vi "Load_LDA_Channel_Setup.vi"(1 "LDA Setup":T1[](array[typedef]) {"Fs" format="%#_pHz"; "syncDelay" format="%#_gms"; "Ch" min=0 step=1}, 2 "Setup file string":string) -> ()   [LabVIEW 2022 SP3]
uses:
  Controls/Meas input Cluster.ctl
  Controls/Inst_type.ctl
  Controls/portOrDev.ctl
  Controls/calType.ctl
  Controls/channelState.ctl
  <vilib>/Utility/error.llb/Trim Whitespace One-Sided.vi
  Globals/LDA_global.vi
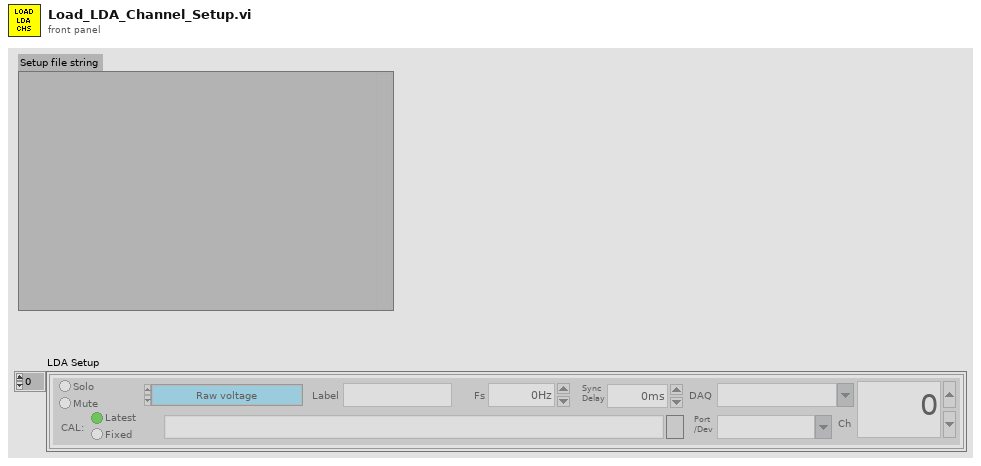
[diagram p1: front panel]
types:
  T1 = typedef "Meas input Cluster.ctl" = cluster{"Type":T2, "Label":string, "DAQ":string, "Port":T3, "Ch":i32, "Cal":path, "calType":T4, "Fs":dbl, "syncDelay":dbl, "chState":T5}
  T2 = typedef "Inst_type.ctl" = enum16{"Raw voltage", "Raw with zero offsetting", "Propeller anemometer", "Pressure Transducer", "Pitot-static tube", "Hot wire", "Cross wire 1", "Cross wire 2", "Generic Linear", "Generic Polynomial", "Generic BackPoly", "Fast FID", "Thermocouple", "Cold wire", "Pulsed Wire", "LDA Vel", "LDA Tran time", "LDA Arr time", "Microphone"}
  T3 = typedef "portOrDev.ctl" = string
  T4 = typedef "calType.ctl" = enum32{"Latest", "Fixed"}
  T5 = typedef "channelState.ctl" = enum32{"No Selection", "Solo", "Mute"}
  T6 = typedef "LDA_Channel.ctl" = cluster{"Wavelength (nm)":dbl, "Vel Comp":string, "Max Velocity":dbl, "Min Velocity":dbl, "Max Record length":u16, "Signal gain (dB)":i16, "High voltage":i16, "Optics Conversion Factor":dbl, "Min Record length":u16, "Multiply Velocity by -1":bool, "Signal to Noise Ratio":string, "Validation Ratio":string, "Probe":string, "Laser":string, "BSA":string, "Lense":string, "Beam Separation (mm)":dbl, "Focal Length (mm)":dbl, "COLOUR":u32, "BSA IP":string, "Velocity Range (m/s)":dbl, "Centre Velocity (m/s)":dbl, "Unshifted mW":dbl, "Shifted mW":dbl, "Bandwidth Hz":dbl, "Req Sampling Rate Hz":dbl, "Ch":i32, "CenterFreq Hz":dbl, "Laser IP":string, "Sync Delay (s)":dbl}
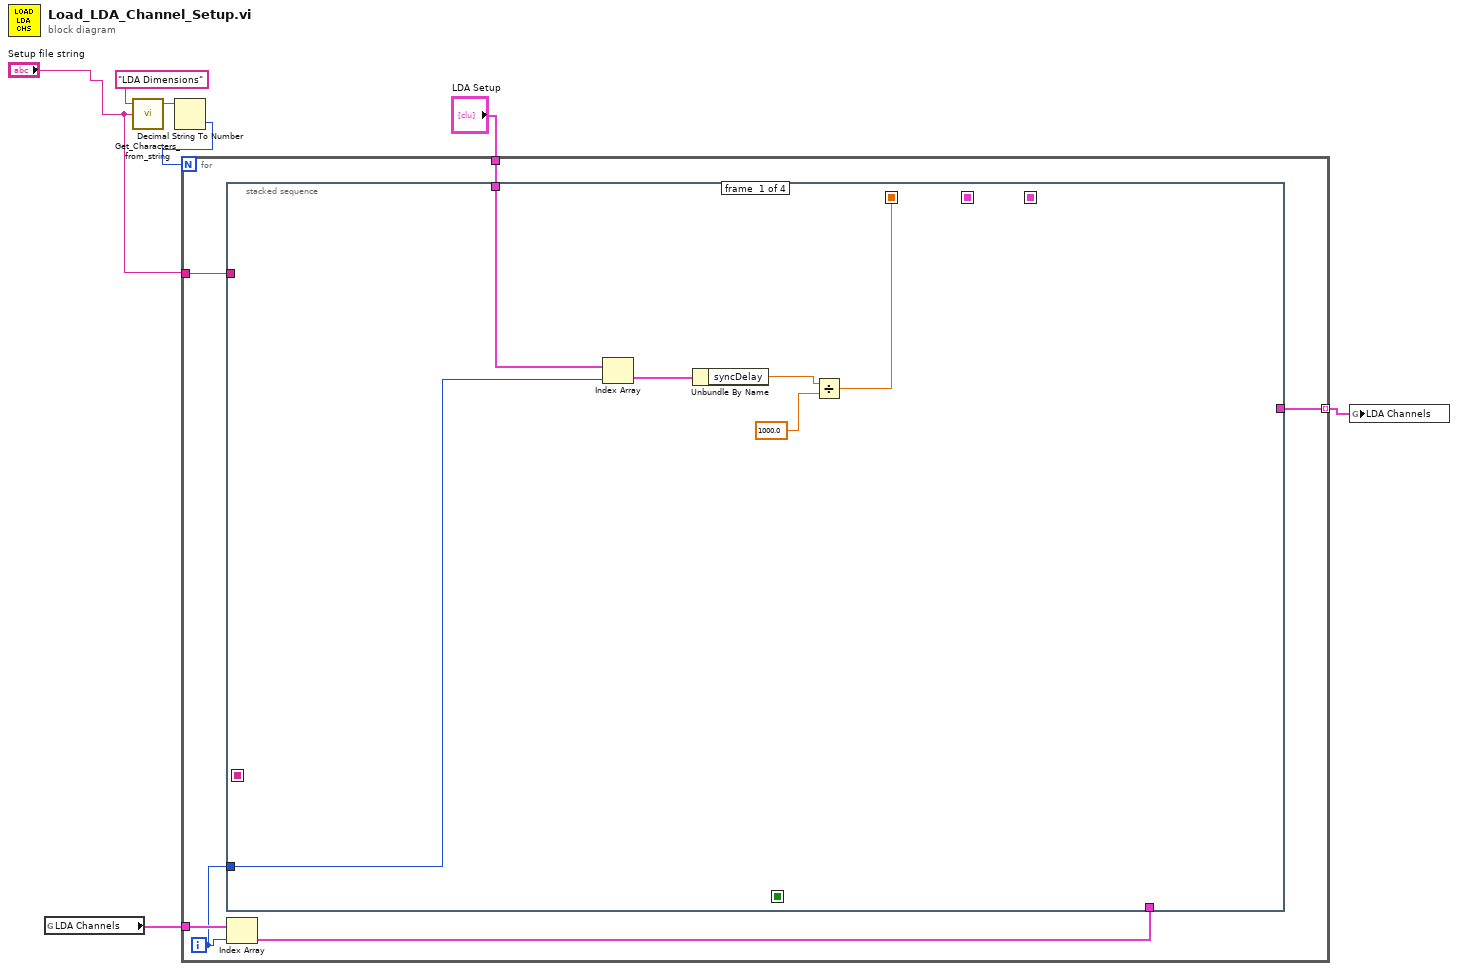
[diagram p0: block diagram]
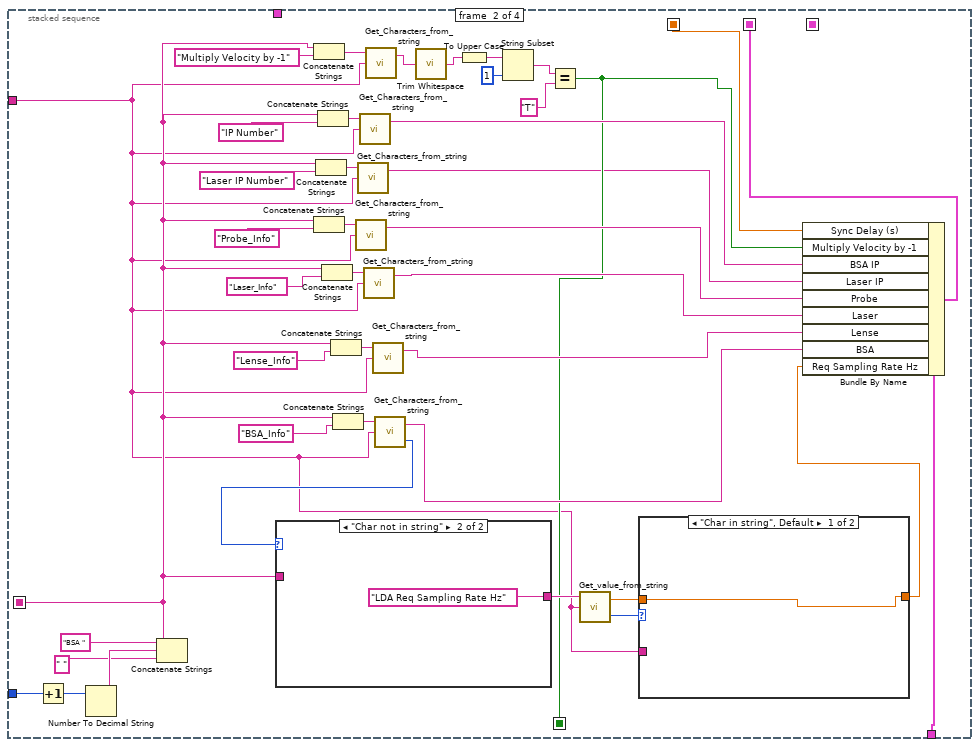
[diagram p2: hidden frame]
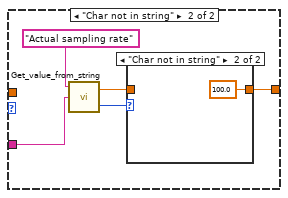
[diagram p3: hidden frame]
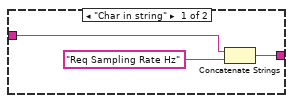
[diagram p5: hidden frame]
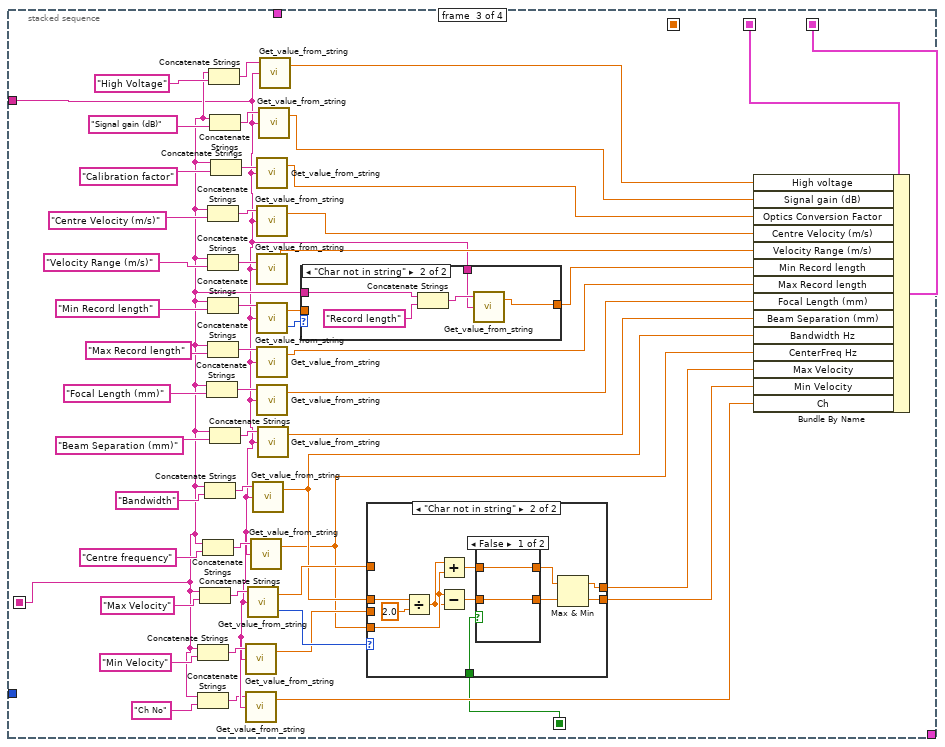
[diagram p6: hidden frame]
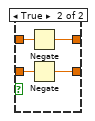
[diagram p8: hidden frame]
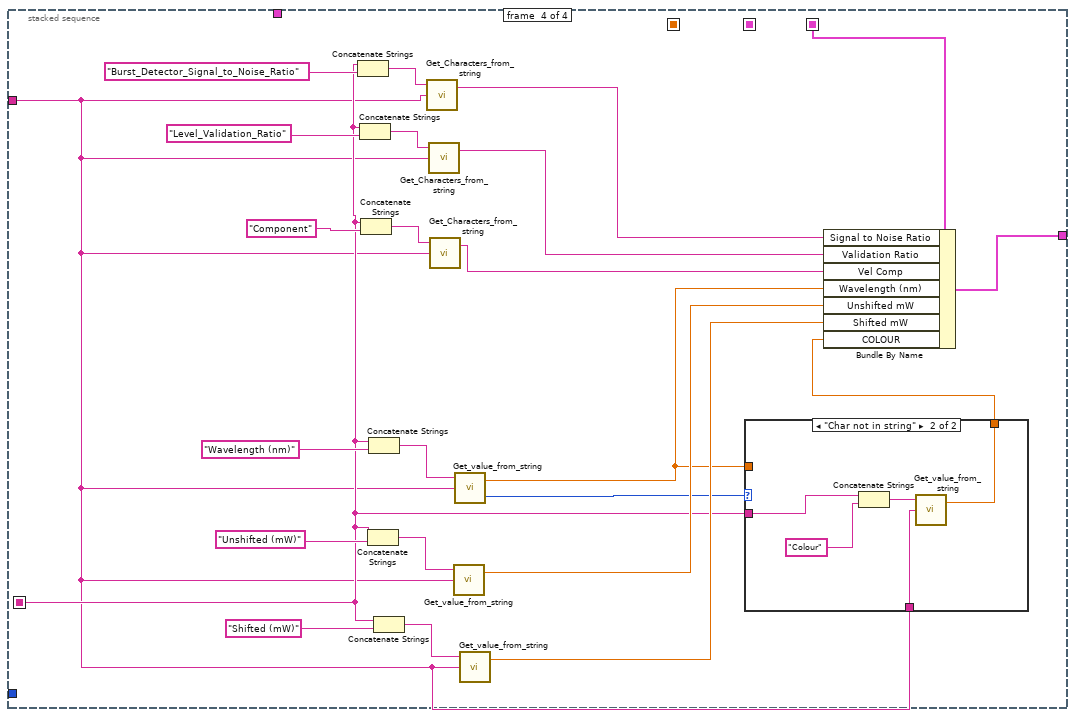
[diagram p10: hidden frame]
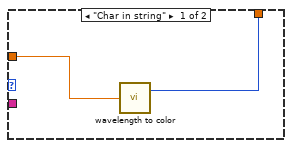
[diagram p11: hidden frame]
diagram:
  n1 = global read "LDA_global.vi" "LDA Channels"() -> (w3:T6[])
  n2 = call "Get_Characters_from_string.vi"("Input string"="Setup file string", "Variable name"="LDA Dimensions") -> ("Value"=w7:string)  [unwired: 1 in, 1 out]
  n3 = Decimal String To Number(string=w7) -> (number=w5:i32)  [unwired: 2 in, 1 out]
  n4 = for {
    N: w5 -> [_]
    tunnel: w3 -> [w13]
    tunnel: "Setup file string" -> [w10]
    tunnel: [w9] -> w2 mode=indexing
    tunnel: "LDA Setup" -> [w8]
    i -> [w12]
    n5 = Index Array(array=w13, index=w12) -> (element=w11:T6)
    n6 = stacked-sequence {
      seq-local: [_ w22 _ _] -> [_ _ w85 w152]
      seq-local: [_ w49 _ _] -> [_ _ w100 _]
      seq-local: [_ _ w99 _] -> [_ _ _ w172]
      seq-local: [_ w26 _ _] -> [_ _ w74 _]
      seq-local: [w14 _ _ _] -> [_ w20 _ _]
      tunnel: w12 -> [w18 w48 _ _]
      tunnel: w11 -> [_ w58 _ _]
      tunnel: w10 -> [_ w21 w84 w151]
      tunnel: [_ _ _ w168] -> w9
      tunnel: w8 -> [w19 _ _ _]
      frame #0 {
        n7 = Index Array(array=w19, index=w18) -> (element=w17:T1)
        n8 = Unbundle By Name(w17) -> ("syncDelay"=w16:dbl)
        n9 = Divide(x=w16, y=1000.0) -> (x/y=w14:dbl)
      }
      frame #1 {
        n10 = Increment(x=w48) -> (x+1=w47:i32)
        n11 = Number To Decimal String(number=w47) -> (decimal integer string=w61:string)  [unwired: 1 out]
        n12 = Concatenate Strings("BSA ", w61, " ") -> (w22:string)
        n13 = Concatenate Strings(w22, "Multiply Velocity by -1") -> (w27:string)
        n14 = Concatenate Strings(w22, "Probe_Info" ("Pre Setup String")) -> (w57:string)
        n15 = Concatenate Strings(w22, "Laser IP Number" ("Pre Setup String")) -> (w24:string)
        n16 = Concatenate Strings(w22, "IP Number" ("Pre Setup String")) -> (w36:string)
        n17 = Concatenate Strings(w22, "Laser_Info" ("string")) -> (w55:string)
        n18 = Concatenate Strings(w22, "Lense_Info" ("string")) -> (w54:string)
        n19 = Concatenate Strings(w22, "BSA_Info" ("string")) -> (w53:string)
        n20 = call "Get_Characters_from_string.vi"("Input string"=w21, "Variable name"=w57) -> ("Value"=w43:string)  [unwired: 1 in, 1 out]
        n21 = call "Get_Characters_from_string.vi"("Input string"=w21, "Variable name"=w24) -> ("Value"=w23:string)  [unwired: 1 in, 1 out]
        n22 = call "Get_Characters_from_string.vi"("Input string"=w21, "Variable name"=w36) -> ("Value"=w35:string)  [unwired: 1 in, 1 out]
        n23 = call "Get_Characters_from_string.vi"("Input string"=w21, "Variable name"=w55) -> ("Value"=w44:string)  [unwired: 1 in, 1 out]
        n24 = call "Get_Characters_from_string.vi"("Input string"=w21, "Variable name"=w27) -> ("Value"=w34:string)  [unwired: 1 in, 1 out]
        n25 = call "Get_Characters_from_string.vi"("Input string"=w21, "Variable name"=w54) -> ("Value"=w45:string)  [unwired: 1 in, 1 out]
        n26 = call "Get_Characters_from_string.vi"("Input string"=w21, "Variable name"=w53) -> ("Status"=w42:enum16{"Char in string", "Char not in string"}, "Value"=w46:string)  [unwired: 1 in]
        n27 = case shown="\"Char not in string\"" w42 {
          tunnel: w22 -> [w71 _]
          tunnel: [w70 "LDA Req Sampling Rate Hz"] -> w41
          frame "Char in string" {
            n28 = Concatenate Strings(w71, "Req Sampling Rate Hz") -> (w70:string)
          }
          frame "Char not in string" {
          }
        }
        n29 = call <vilib>:"Trim Whitespace.vi"("string"=w34) -> ("trimmed string"=w33:string)  [unwired: 1 in]
        n30 = To Upper Case(1:w33) -> (0:w32:string)
        n31 = String Subset(string=w32, length (rest)=1 ("length (rest)")) -> (substring=w30:string)  [unwired: 1 in]
        n32 = Equal?(x=w30, y="T") -> (x = y?=w26:bool)
        n33 = call "Get_value_from_string.vi"("Input string"=w21, "Variable name"=w41) -> ("Status"=w40:enum16{"Char in string", "Char not in string"}, "Value"=w38:dbl)  [unwired: 1 in]
        n34 = case shown="\"Char in string\", Default" w40 {
          tunnel: w21 -> [_ w66]
          tunnel: [w62 w64] -> w39
          tunnel: w38 -> [w62 _]
          frame "Char in string", Default {
          }
          frame "Char not in string" {
            n35 = call "Get_value_from_string.vi"("Input string"=w66, "Variable name"="Actual sampling rate") -> ("Status"=w65:enum16{"Char in string", "Char not in string"}, "Value"=w63:dbl)  [unwired: 1 in]
            n36 = case shown="\"Char not in string\"" w65 {
              tunnel: [w68 100.0 ("Value")] -> w64
              tunnel: w63 -> [w68 _]
              frame "Char in string" {
              }
              frame "Char not in string" {
              }
            }
          }
        }
        n37 = Bundle By Name(cluster=w58, "Sync Delay (s)"=w20, "Multiply Velocity by -1"=w26, "BSA IP"=w35, "Laser IP"=w23, "Probe"=w43, "Laser"=w44, "Lense"=w45, "BSA"=w46, "Req Sampling Rate Hz"=w39) -> (w49:T6)
      }
      frame #2 {
        n38 = Concatenate Strings(w85, "Min Velocity" ("Label for characters")) -> (w88:string)
        n39 = Concatenate Strings(w85, "Ch No" ("Label for characters")) -> (w83:string)
        n40 = Concatenate Strings(w85, "Max Velocity" ("Label for characters")) -> (w87:string)
        n41 = Concatenate Strings(w85, "Centre frequency" ("Label for characters")) -> (w96:string)
        n42 = Concatenate Strings(w85, "Bandwidth" ("Label for characters")) -> (w97:string)
        n43 = Concatenate Strings(w85, "Focal Length (mm)" ("Label for characters")) -> (w123:string)
        n44 = Concatenate Strings(w85, "Centre Velocity (m/s)") -> (w113:string)
        n45 = Concatenate Strings(w85, "Velocity Range (m/s)") -> (w114:string)
        n46 = Concatenate Strings(w85, "Min Record length") -> (w115:string)
        n47 = Concatenate Strings(w85, "Max Record length") -> (w120:string)
        n48 = Concatenate Strings(w85, "High Voltage") -> (w119:string)
        n49 = Concatenate Strings(w85, "Signal gain (dB)") -> (w118:string)
        n50 = Concatenate Strings(w85, "Beam Separation (mm)" ("Label for characters")) -> (w122:string)
        n51 = Concatenate Strings(w85, "Calibration factor") -> (w112:string)
        n52 = call "Get_value_from_string.vi"("Input string"=w84, "Variable name"=w88) -> ("Value"=w77:dbl)  [unwired: 1 in, 1 out]
        n53 = call "Get_value_from_string.vi"("Input string"=w84, "Variable name"=w83) -> ("Value"=w82:dbl)  [unwired: 1 in, 1 out]
        n54 = call "Get_value_from_string.vi"("Input string"=w84, "Variable name"=w87) -> ("Status"=w81:enum16{"Char in string", "Char not in string"}, "Value"=w79:dbl)  [unwired: 1 in]
        n55 = call "Get_value_from_string.vi"("Input string"=w84, "Variable name"=w96) -> ("Value"=w75:dbl)  [unwired: 1 in, 1 out]
        n56 = call "Get_value_from_string.vi"("Input string"=w84, "Variable name"=w97) -> ("Value"=w76:dbl)  [unwired: 1 in, 1 out]
        n57 = call "Get_value_from_string.vi"("Input string"=w84, "Variable name"=w112) -> ("Value"=w103:dbl)  [unwired: 1 in, 1 out]
        n58 = call "Get_value_from_string.vi"("Input string"=w84, "Variable name"=w113) -> ("Value"=w104:dbl)  [unwired: 1 in, 1 out]
        n59 = call "Get_value_from_string.vi"("Input string"=w84, "Variable name"=w114) -> ("Value"=w105:dbl)  [unwired: 1 in, 1 out]
        n60 = call "Get_value_from_string.vi"("Input string"=w84, "Variable name"=w115) -> ("Status"=w93:enum16{"Char in string", "Char not in string"}, "Value"=w91:dbl)  [unwired: 1 in]
        n61 = call "Get_value_from_string.vi"("Input string"=w84, "Variable name"=w120) -> ("Value"=w98:dbl)  [unwired: 1 in, 1 out]
        n62 = call "Get_value_from_string.vi"("Input string"=w84, "Variable name"=w123) -> ("Value"=w106:dbl)  [unwired: 1 in, 1 out]
        n63 = call "Get_value_from_string.vi"("Input string"=w84, "Variable name"=w122) -> ("Value"=w107:dbl)  [unwired: 1 in, 1 out]
        n64 = call "Get_value_from_string.vi"("Input string"=w84, "Variable name"=w118) -> ("Value"=w102:dbl)  [unwired: 1 in, 1 out]
        n65 = call "Get_value_from_string.vi"("Input string"=w84, "Variable name"=w119) -> ("Value"=w101:dbl)  [unwired: 1 in, 1 out]
        n66 = case shown="\"Char not in string\"" w93 {
          tunnel: [w145 w146] -> w92
          tunnel: w91 -> [w145 _]
          tunnel: w85 -> [_ w150]
          tunnel: w84 -> [_ w147]
          frame "Char in string" {
          }
          frame "Char not in string" {
            n67 = Concatenate Strings(w150, "Record length") -> (w148:string)
            n68 = call "Get_value_from_string.vi"("Input string"=w147, "Variable name"=w148) -> ("Value"=w146:dbl)  [unwired: 1 in, 1 out]
          }
        }
        n69 = case shown="\"Char not in string\"" w81 {
          tunnel: [w127 w129] -> w80
          tunnel: w79 -> [w127 _]
          tunnel: [w126 w128] -> w78
          tunnel: w77 -> [w126 _]
          tunnel: w76 -> [_ w138]
          tunnel: w75 -> [_ w136]
          tunnel: w74 -> [_ w134]
          frame "Char in string" {
          }
          frame "Char not in string" {
            n70 = Divide(x=w138, y=2.0) -> (x/y=w135:dbl)
            n71 = Add(x=w135, y=w136) -> (x+y=w133:dbl)
            n72 = Subtract(x=w136, y=w135) -> (x-y=w132:dbl)
            n73 = case shown="False" w134 {
              tunnel: w133 -> [w140 w144]
              tunnel: w132 -> [w139 w143]
              tunnel: [w140 w142] -> w131
              tunnel: [w139 w141] -> w130
              frame False {
              }
              frame True {
                n74 = Negate(x=w144) -> (-x=w142:dbl)
                n75 = Negate(x=w143) -> (-x=w141:dbl)
              }
            }
            n76 = Max & Min(x=w131, y=w130) -> (max(x,y)=w129:dbl, min(x,y)=w128:dbl)
          }
        }
        n77 = Bundle By Name(cluster=w100, "High voltage"=w101, "Signal gain (dB)"=w102, "Optics Conversion Factor"=w103, "Centre Velocity (m/s)"=w104, "Velocity Range (m/s)"=w105, "Min Record length"=w92, "Max Record length"=w98, "Focal Length (mm)"=w106, "Beam Separation (mm)"=w107, "Bandwidth Hz"=w76, "CenterFreq Hz"=w75, "Max Velocity"=w80, "Min Velocity"=w78, "Ch"=w82) -> (w99:T6)
      }
      frame #3 {
        n78 = Concatenate Strings(w152, "Burst_Detector_Signal_to_Noise_Ratio" ("Pre Setup String")) -> (w161:string)
        n79 = Concatenate Strings(w152, "Level_Validation_Ratio" ("Pre Setup String")) -> (w160:string)
        n80 = Concatenate Strings(w152, "Component") -> (w173:string)
        n81 = Concatenate Strings(w152, "Unshifted (mW)") -> (w167:string)
        n82 = Concatenate Strings(w152, "Wavelength (nm)") -> (w170:string)
        n83 = Concatenate Strings(w152, "Shifted (mW)") -> (w166:string)
        n84 = call "Get_Characters_from_string.vi"("Input string"=w151, "Variable name"=w161) -> ("Value"=w156:string)  [unwired: 1 in, 1 out]
        n85 = call "Get_Characters_from_string.vi"("Input string"=w151, "Variable name"=w160) -> ("Value"=w157:string)  [unwired: 1 in, 1 out]
        n86 = call "Get_Characters_from_string.vi"("Input string"=w151, "Variable name"=w173) -> ("Value"=w169:string)  [unwired: 1 in, 1 out]
        n87 = call "Get_value_from_string.vi"("Input string"=w151, "Variable name"=w167) -> ("Value"=w163:dbl)  [unwired: 1 in, 1 out]
        n88 = call "Get_value_from_string.vi"("Input string"=w151, "Variable name"=w170) -> ("Status"=w155:enum16{"Char in string", "Char not in string"}, "Value"=w154:dbl)  [unwired: 1 in]
        n89 = call "Get_value_from_string.vi"("Input string"=w151, "Variable name"=w166) -> ("Value"=w162:dbl)  [unwired: 1 in, 1 out]
        n90 = case shown="\"Char not in string\"" w155 {
          tunnel: w154 -> [w176 _]
          tunnel: [w175 w178] -> w153
          tunnel: w152 -> [_ w179]
          tunnel: w151 -> [_ w177]
          frame "Char in string" {
            n91 = call "wavelength to color.vi"("Wavelength (380 - 780)"=w176) -> ("Color"=w175:u32)  [unwired: 1 out]
          }
          frame "Char not in string" {
            n92 = Concatenate Strings(w179, "Colour") -> (w181:string)
            n93 = call "Get_value_from_string.vi"("Input string"=w177, "Variable name"=w181) -> ("Value"=w178:dbl)  [unwired: 1 in, 1 out]
          }
        }
        n94 = Bundle By Name(cluster=w172, "Signal to Noise Ratio"=w156, "Validation Ratio"=w157, "Vel Comp"=w169, "Wavelength (nm)"=w154, "Unshifted mW"=w163, "Shifted mW"=w162, "COLOUR"=w153) -> (w168:T6)
      }
    }
  }
  n95 = global write "LDA_global.vi" "LDA Channels"(w2) -> ()
